vi "Measurements.vi"(8 "error in (no error)":errorcluster, 10 "Variant":variant, 11 "Module":refnum<class "ModuleAdmin.lvclass">) -> (0 "error out":errorcluster)   [LabVIEW 2018, in "AcPwrPlugins.lvlib"]
doc: "This VI broadcasts the instrument's measurements."
uses:
  AcPwrPlugins.lvlib
  <userlib>/NIST/ModuleAdminLib/ModuleAdmin/ModuleAdmin.lvclass
  AcPwrShared/clEventType.ctl
  AcPwrShared/AcPwrShared.lvlib
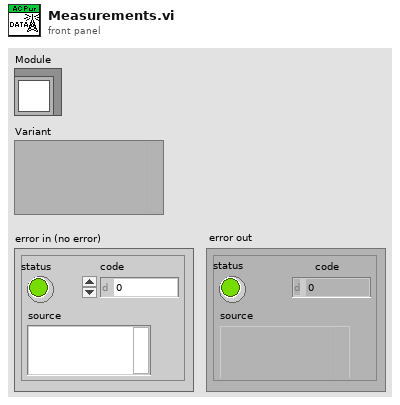
[diagram p1: front panel]
types:
  T1 = typedef "AcPwrShared.lvlib/clEventType.ctl" = cluster{"ModuleID":i32, "Data":variant}
  T2 = typedef "AcPwrShared.lvlib/AcPwrBroadcastEvents.ctl" = cluster{"DidInit":refnum<user-event>, "StatusUpdate":refnum<user-event>, "ErrorReport":refnum<user-event>, "DidStop":refnum<user-event>, "PathToINI":refnum<user-event>, "Measurements":refnum<user-event>, "LoadConfigFile":refnum<user-event>, "GetSettings":refnum<user-event>, "SetSettings":refnum<user-event>, "GetType&ID":refnum<user-event>, "GotSettings":refnum<user-event>, "GotSettingsLV":refnum<user-event>}
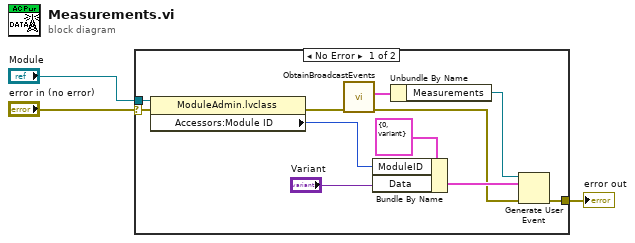
[diagram p0: block diagram]
diagram:
  n1 = case shown="No Error" "error in (no error)" {
    selector: "error in (no error)" -> [w14 w15]
    tunnel: "Module" -> [w13 _]
    tunnel: [w12 w15] -> w1
    frame No Error {
      n2 = property class="ModuleAdmin.lvclass"(reference=w13, error in=w14) -> (error out=w5:errorcluster, "Accessors:Module ID"=w11:i32)  [unwired: 1 out]
      n3 = call "ObtainBroadcastEvents.vi"("error in (no error)"=w5) -> ("error out"=w6:errorcluster, "AcPwrEvents"=w8:T2)  [unwired: 9 in]
      n4 = Bundle By Name(cluster=T1 {"ModuleID"=0, "Data"=variant} ("clEventType"), "ModuleID"=w11, "Data"="Variant") -> (w9:T1)
      n5 = Unbundle By Name(w8) -> ("Measurements"=w7:refnum<user-event>)
      n6 = Generate User Event(user event=w7, event data cluster=w9, error in=w6) -> (error out=w12:errorcluster)  [unwired: 1 in, 1 out]
    }
    frame Error {
    }
  }
  "error out" <- w1
